vi "Configure Cache.vi"(8 "error in (no error)":errorcluster, 9 "Cache Size":i32=128 format="%.0x", 11 "navX Registry Cache in":refnum<class "navX Registry Cache.lvclass">) -> (0 "error out":errorcluster, 3 "navX Registry Cache out":refnum<class "navX Registry Cache.lvclass">)   [LabVIEW 2015, in "navX Library v3.lvlib" / "navX Registry Cache.lvclass"]
uses:
  navX Registry Cache.lvclass
  navX Registry Cache.lvclass/navX Registry Cache.ctl
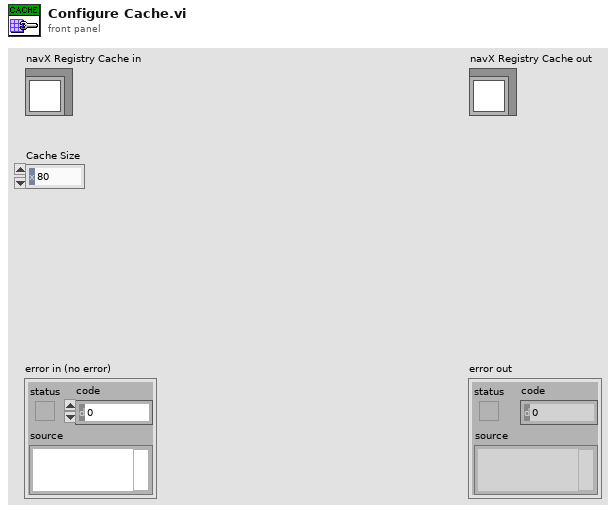
[diagram p1: front panel]
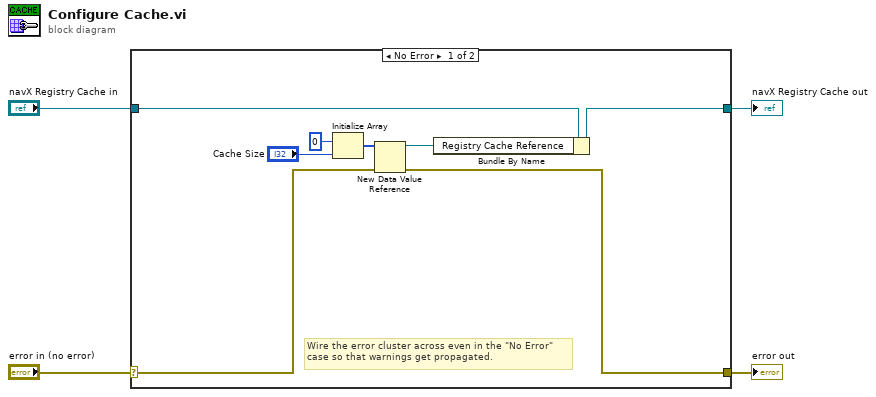
[diagram p0: block diagram]
diagram:
  n1 = case shown="No Error" "error in (no error)" {
    selector: "error in (no error)" -> [w6 w14]
    tunnel: [w5 w14] -> w3
    tunnel: [w11 w13] -> w1
    tunnel: "navX Registry Cache in" -> [w12 w13]
    frame No Error {
      # "Wire the error cluster across even in the \"No Error\"\ncase so that warnings get propagated."
      n2 = Initialize Array(u8 0, "Cache Size") -> (w9:u8[])
      n3 = New Data Value Reference(data value=w9, error in=w6) -> (data value reference=w7:refnum<data-value>, error out=w5:errorcluster)
      n4 = Bundle By Name(cluster=w12, "Registry Cache Reference"=w7) -> (w11:refnum<class "navX Registry Cache.lvclass">)
    }
    frame Error {
    }
  }
  "error out" <- w3
  "navX Registry Cache out" <- w1
